vi "uC_connect.vi"(10 "reference":refnum<visa-resource-name>, 11 "find port":bool) -> (0 "+":dbl, 1 "C":dbl, 2 "B":dbl, 3 "A":dbl, 4 "=":dbl, 5 "VISA resource name out":refnum<visa-resource-name>, 6 "status":bool, 7 "String":string)   [LabVIEW 2020]
uses:
  <vilib>/Instr/_visa.llb/VISA Find Search Mode.ctl
panel:
  out "Array":string[](array[string])
  out "read buffer":string
  out "source":string
  out "code":i32
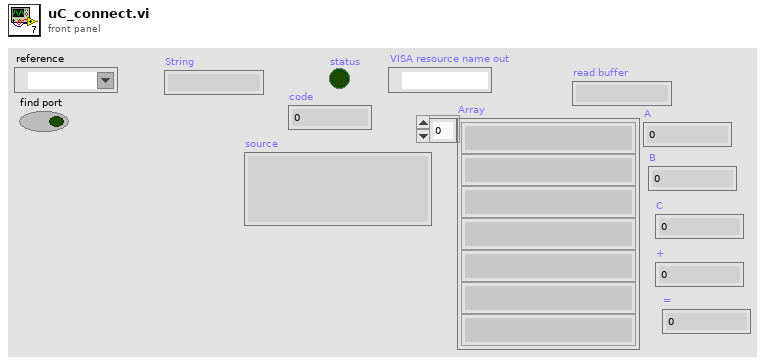
[diagram p1: front panel]
types:
  T1 = typedef "VISA Find Search Mode.ctl" = u32
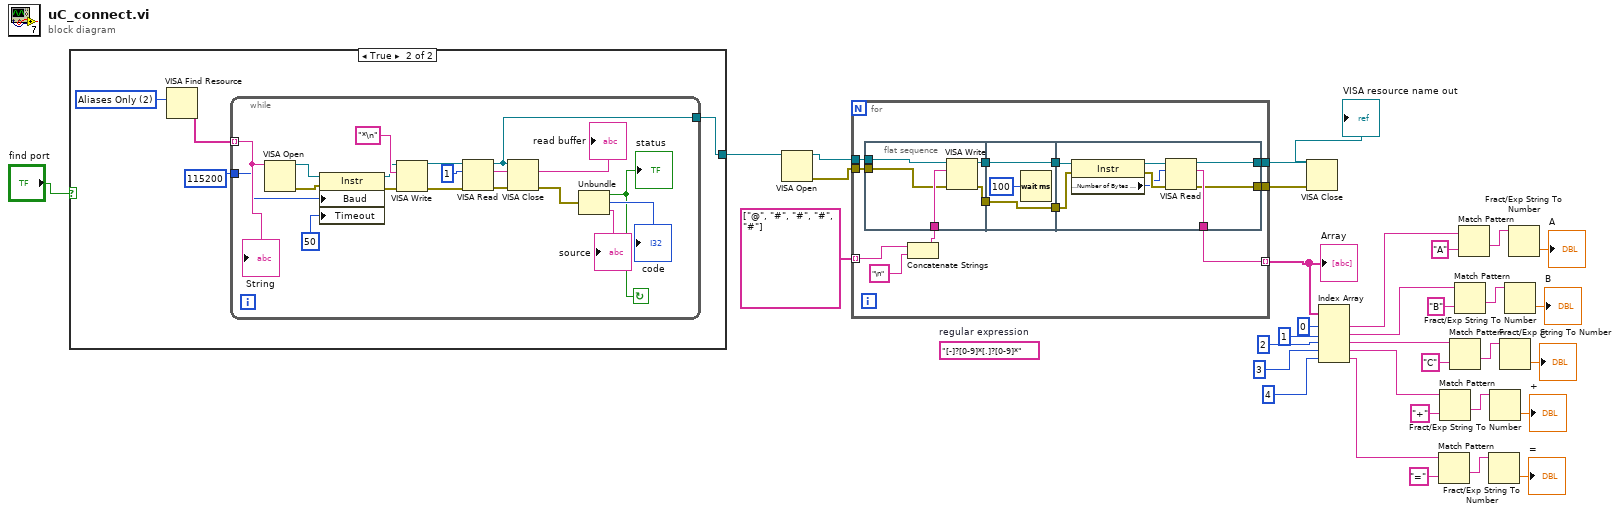
[diagram p0: block diagram]
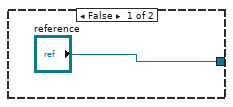
[diagram p2: hidden frame]
diagram:
  (unwired) "[-]?[0-9]*[.]?[0-9]*"  # regular expression
  n1 = case shown="True" "find port" {
    tunnel: ["reference" w38] -> w30
    frame False {
    }
    frame True {
      w37 = T1 2 items=["Canonical Names Only"=0, "Aliases Only"=2, "Include Matching Aliases"=3, "Include All Aliases"=4] ("Search Mode")
      n2 = VISA Find Resource(10:w37) -> (3:w35:string[])  [unwired: 2 in, 2 out]
      n3 = while {
        tunnel: w35 -> [w45] mode=indexing
        tunnel: u32 115200 ("baud rate (9600)") -> [w40]
        tunnel: [w46] -> w38
        stop <- w49 continue-if-true
        n4 = VISA Open(VISA resource name=w45) -> (VISA resource name=w44:refnum<visa-resource-name>, error out=w42:errorcluster)  [unwired: 4 in]
        n5 = property class="Instr"(reference=w44, error in=w42, "Baud"=w40, "Timeout"=u32 50 ("timeout (10sec)")) -> (reference out=w43:refnum<visa-resource-name>, error out=w41:errorcluster)
        n6 = VISA Write(VISA resource name=w43, write buffer="*\n", error in (no error)=w41) -> (VISA resource name out=w54:refnum<visa-resource-name>, error out=w55:errorcluster)  [unwired: 1 out]
        n7 = VISA Read(VISA resource name=w54, byte count=u32 1, error in (no error)=w55) -> (VISA resource name out=w46:refnum<visa-resource-name>, read buffer=→"read buffer":string, error out=w48:errorcluster)  [unwired: 1 out]
        n8 = VISA Close(VISA resource name=w46, error in (no error)=w48) -> (error out=w47:errorcluster)
        n9 = Unbundle(w47) -> ("status"=w49:bool, "code"=→"code":i32, "source"=→"source":string)
        "status" <- w49
        "String" <- w45
      }
    }
  }
  n10 = VISA Open(VISA resource name=w30) -> (VISA resource name=w31:refnum<visa-resource-name>, error out=w32:errorcluster)  [unwired: 4 in]
  n11 = for {
    tunnel: string[] ["@", "#", "#", "#", "#"] -> [w67] mode=indexing
    tunnel: [w61] -> w27 mode=indexing
    tunnel: w32 -> [w60]
    tunnel: w31 -> [w59]
    tunnel: [w58] -> w29
    tunnel: [w57] -> w28
    n12 = flat-sequence {
      tunnel: w68 -> [w73]
      tunnel: [w72] -> w64
      tunnel: [w71] -> w63
      tunnel: w60 -> [w70]
      tunnel: w59 -> [w69]
      tunnel: [w75] -> w65
      tunnel: w64 -> [w75]
      tunnel: w63 -> [w74]
      tunnel: [w74] -> w62
      tunnel: w65 -> [w84]
      tunnel: w62 -> [w80]
      tunnel: [w79] -> w61
      tunnel: [w78] -> w58
      tunnel: [w77] -> w57
      frame #0 {
        n13 = VISA Write(VISA resource name=w69, write buffer=w73, error in (no error)=w70) -> (VISA resource name out=w72:refnum<visa-resource-name>, error out=w71:errorcluster)  [unwired: 1 out]
      }
      frame #1 {
        n14 = Wait (ms)(milliseconds to wait=u32 100) -> ()  [unwired: 1 out]
      }
      frame #2 {
        n15 = property class="Instr"(reference=w84, error in=w80) -> (reference out=w83:refnum<visa-resource-name>, error out=w82:errorcluster, "Serial Settings:Number of Bytes at Serial Port"=w81:u32)
        n16 = VISA Read(VISA resource name=w83, byte count=w81, error in (no error)=w82) -> (VISA resource name out=w77:refnum<visa-resource-name>, read buffer=w79:string, error out=w78:errorcluster)  [unwired: 1 out]
      }
    }
    n17 = Concatenate Strings(w67, "\n") -> (w68:string)
  }
  "Array" <- w27
  "VISA resource name out" <- w28
  n18 = VISA Close(VISA resource name=w28, error in (no error)=w29) -> ()  [unwired: 1 out]
  n19 = Index Array(array=w27, index #1=0 ("index"), index #2=1 ("index"), index #3=2 ("index"), index #4=3 ("index"), index #5=4 ("index")) -> (element #1=w6:string, element #2=w5:string, element #3=w4:string, element #4=w3:string, element #5=w2:string)
  n20 = Match Pattern(string=w2, regular expression="=") -> (after substring=w7:string)  [unwired: 1 in, 3 out]
  n21 = Match Pattern(string=w3, regular expression="+") -> (after substring=w10:string)  [unwired: 1 in, 3 out]
  n22 = Match Pattern(string=w4, regular expression="C") -> (after substring=w13:string)  [unwired: 1 in, 3 out]
  n23 = Match Pattern(string=w5, regular expression="B") -> (after substring=w16:string)  [unwired: 1 in, 3 out]
  n24 = Match Pattern(string=w6, regular expression="A") -> (after substring=w23:string)  [unwired: 1 in, 3 out]
  n25 = Fract/Exp String To Number(string=w7) -> (number=→"=":dbl)  [unwired: 3 in, 1 out]
  n26 = Fract/Exp String To Number(string=w10) -> (number=→"+":dbl)  [unwired: 3 in, 1 out]
  n27 = Fract/Exp String To Number(string=w13) -> (number=→"C":dbl)  [unwired: 3 in, 1 out]
  n28 = Fract/Exp String To Number(string=w16) -> (number=→"B":dbl)  [unwired: 3 in, 1 out]
  n29 = Fract/Exp String To Number(string=w23) -> (number=→"A":dbl)  [unwired: 3 in, 1 out]
